vi "permut_comb_fact_MAIN.vi"() -> ()   [LabVIEW 2026]
panel:
  out "n!/(n-r)!":dbl
  in  "r":dbl
  in  "(n)":dbl
  in  "n!":dbl
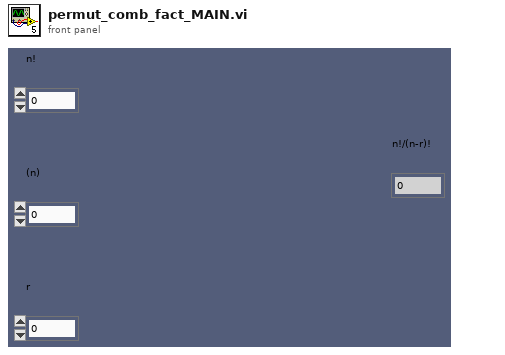
[diagram p1: front panel]
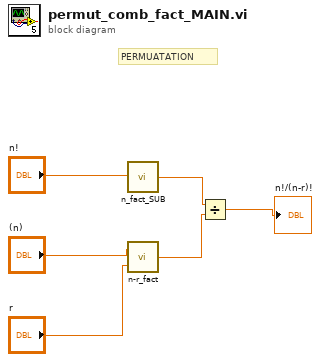
[diagram p0: block diagram]
diagram:
  # "PERMUATATION"
  n1 = call "n_fact_SUB.vi"("n"="n!") -> ("n!"=w3:dbl)
  n2 = call "n-r_fact.vi"("r"="r", "n"="(n)") -> ("(n-r)!"=w2:dbl)
  n3 = Divide(x=w3, y=w2) -> (x/y=→"n!/(n-r)!":dbl)
